vi "SendPacket.vi"(6 "timeout (0ms : no ack)":i32, 8 "error in (no error)":errorcluster, 10 "ControlPacket":refnum<class "ControlPacket.lvclass">, 11 "Client in":refnum<class "Client.lvclass">) -> (0 "error out":errorcluster, 2 "Response":refnum<class "ControlPacket.lvclass">[](array[class]), 3 "Client out":refnum<class "Client.lvclass">)   [LabVIEW 2013, in "MQTT Server.lvlib" / "Client.lvclass"]
uses:
  Client.lvclass
  Control Packets/ControlPacket/ControlPacket.lvclass
  Client.lvclass/Client.ctl
  Control Packets/ControlPacket/ControlPacket.lvclass/ControlPacket.ctl
  Server/Session/Session.lvclass
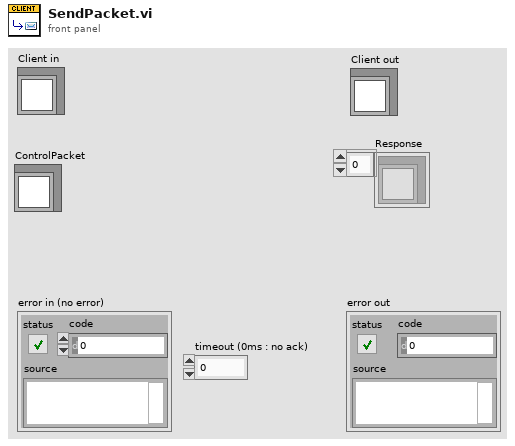
[diagram p1: front panel]
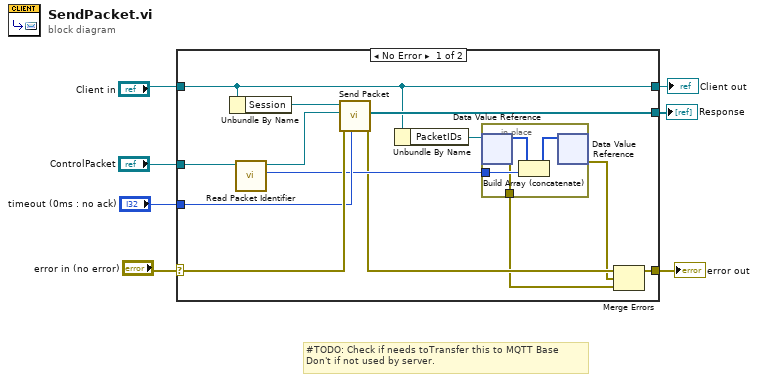
[diagram p0: block diagram]
diagram:
  # "#TODO: Check if needs toTransfer this to MQTT Base\nDon't if not used by server."
  n1 = case shown="No Error" "error in (no error)" {
    selector: "error in (no error)" -> [w19 w26]
    tunnel: [w10 w26] -> w4
    tunnel: [w15 w25] -> w5
    tunnel: "Client in" -> [w15 w25]
    tunnel: "ControlPacket" -> [w17 _]
    tunnel: [w18 _] -> w2
    tunnel: "timeout (0ms : no ack)" -> [w13 _]
    frame No Error {
      n2 = Unbundle By Name(w15) -> ("Session"=w20:refnum<class "Session.lvclass">)
      n3 = call "Read Packet Identifier.vi"("ControlPacket in"=w17) -> ("Packet Identifier"=w12:u16, "ControlPacket out"=w16:refnum<class "ControlPacket.lvclass">)  [unwired: 9 in]
      n4 = call "Send Packet.vi"("timeout (0ms : no ack)"=w13, "error in (no error)"=w19, "Packet"=w16, "Session in"=w20) -> ("error out"=w11:errorcluster, "Response"=w18:refnum<class "ControlPacket.lvclass">[])  [unwired: 4 in, 2 out]
      n5 = Unbundle By Name(w15) -> ("PacketIDs"=w14:refnum<data-value>)
      n6 = in-place {
        in-place-border: w12 -> [w24]
        in-place-border: [w21] -> w8
        n7 = in-place-dvr #1(w14) -> (w23:u16[], w21:errorcluster)
        n8 = Build Array (concatenate)(w23, w24) -> (w22:u16[])
        n9 = in-place-dvr #1(w22) -> (w9:errorcluster)  [unwired: 1 out]
      }
      n10 = Merge Errors(w11, w9, w8) -> (w10:errorcluster)
    }
    frame Error {
    }
  }
  "error out" <- w4
  "Client out" <- w5
  "Response" <- w2
